vi "delta 0.1+7001.vi"() -> ()   [LabVIEW 2019]
uses:
  lib/Keithley 622x/Configure/Format/Typedefs/KE622x -- Results Format.ctl
  lib/Keithley 622x/Configure/Format/Typedefs/KE622x -- Optional Meas Elements.ctl
  lib/Keithley 622x/Configure/Delta PDelta DCon Modes/Typedefs/KE622x -- Delta Mode Params.ctl
  lib/Keithley 622x/Configure/Delta PDelta DCon Modes/Low Level/Typedefs/KE622x -- Delta PDelta Mode High Level.ctl
  lib/Keithley 622x/Configure/Delta PDelta DCon Modes/Low Level/Typedefs/KE622x -- Delta PDelta Mode Low Level.ctl
  lib/Keithley 622x/Configure/Delta PDelta DCon Modes/Low Level/Typedefs/KE622x -- Delta DCon Mode Delay.ctl
  lib/Keithley 622x/Configure/Delta PDelta DCon Modes/Low Level/Typedefs/KE622x -- Delta PDelta Mode Num Cycles Mode.ctl
  lib/Keithley 622x/Configure/Delta PDelta DCon Modes/Low Level/Typedefs/KE622x -- Delta PDelta Mode Num Cycles.ctl
  lib/Keithley 622x/Configure/2182 -A/Low Level/Typedefs/KE2182 -- Voltage Ranges.ctl
  lib/Keithley 622x/Configure/2182 -A/Low Level/Typedefs/KE2182 -- Filter Type.ctl
  lib/Keithley 622x/Configure/2182 -A/Low Level/Typedefs/KE2182 -- Filter Count.ctl
  lib/Keithley 622x/Configure/2182 -A/Low Level/Typedefs/KE2182 -- Filter Window.ctl
  lib/Keithley 622x/Configure/2182 -A/Low Level/Typedefs/KE2182 -- NPLCs.ctl
  lib/Keithley 622x/Configure/Units/Typedefs/KE622x -- Voltage Meas Units.ctl
  KE7001.LLB/Keith 7001 Open/Close Chan.vi
  <vilib>/Utility/file.llb/Write Delimited Spreadsheet (DBL).vi
  lib/Keithley 622x/Keithley 622x.lvlib
panel:
  in  "Meas Units":T1=enum."Ohms"
  out "XY图":cluster{dbl[], dbl[]}(graph)
  in  "file path (dialog if empty)":path caption="文件路径 （空时为对话框）"
  in  "622x Resource":refnum<visa-resource-name>
  in  "Check For SCPI Errors? (T)":bool=TRUE
  in  "2182/2182A Delta Mode Meas Params":T7={"Auto Range?"=TRUE, "Man / Selected\nRange"=enum."10mV", "Enable Digital\nFilter?"=FALSE, "Filter Type"=enum."Moving", "Filter Count"=10, "Filter\nWindow (%)"=0.01, "Enable Analog\nFilter?"=FALSE, "NPLCs"=5} {"Filter\nWindow (%)" min=0.0 max=10.0 step=0.01 format="%.2f"; "Filter Count" min=1 max=100; "NPLCs" min=1 max=10}
  in  "622x Delta Meas Mode Params":T8={"High Level (A)"=0.001, "Low Level (A)"=-0.001, "Delay (s)"=0.002, "Num Cycles Mode"=enum."Finite Count", "Finite Count"=10, "Abort On\nCompliance?"=FALSE, "Cold Swithing\nMode Enabled?"=FALSE} {"Finite Count" min=2 max=65536; "Low Level (A)" min=-0.105 max=0.0 format="%.3p"; "High Level (A)" min=0.0 max=0.105 format="%.3p"; "Delay (s)" min=0.001 max=9999.999 format="%.3f"}
  in  "Meas Timeout\n(msecs)":u32=20000
  out "Execution Time\n(secs)":dbl
  out "Meas\nTimeout?":bool
  in  "Meas Elements To Return":T14={"Timstamp?"=TRUE, "Reading Num?"=TRUE, "Source Value?"=TRUE, "Compliance?"=TRUE, "Average Voltage?"=TRUE}
  in  "Results Format":T15={"Results Format"=enum."Single Prec Bin", "Bin Byte Order"=enum."Swapped"}
  in  "Instrument Type":i32(ring)=3 items=["PPMS", "VersaLab", "DynaCool", "SVSM"]
  # "*** NOTE:  \"Average Voltage\"\nis only available for Differential\nConductance measurements."
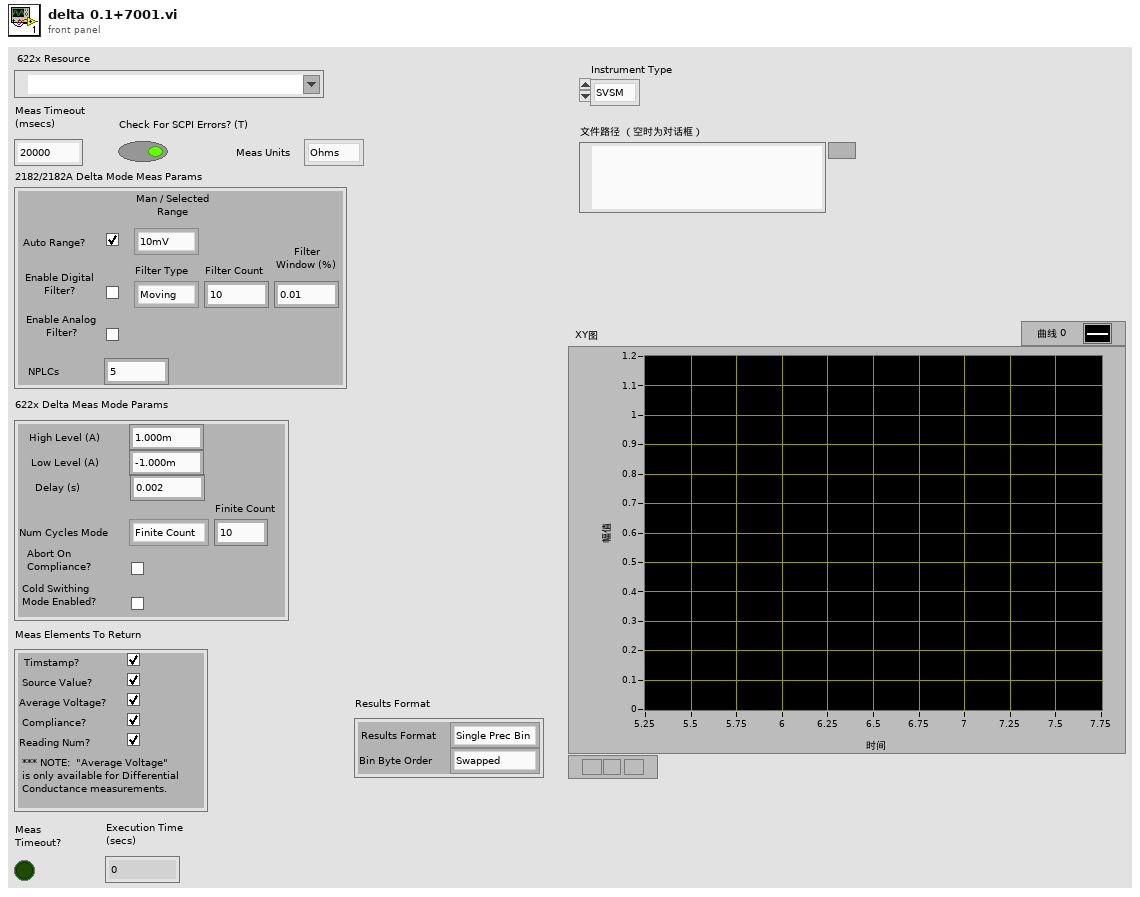
[diagram p1: front panel]
types:
  T1 = typedef "Keithley 622x.lvlib/KE622x -- Voltage Meas Units.ctl" = enum16{"Volts", "Ohms", "Watts", "Siemens"}
  T2 = typedef "Keithley 622x.lvlib/KE2182 -- Voltage Ranges.ctl" = enum16{"10mV", "100mV", "1V", "10V", "100V"}
  T3 = typedef "Keithley 622x.lvlib/KE2182 -- Filter Type.ctl" = enum16{"Moving", "Repeat"}
  T4 = typedef "Keithley 622x.lvlib/KE2182 -- Filter Count.ctl" = u32
  T5 = typedef "Keithley 622x.lvlib/KE2182 -- Filter Window.ctl" = dbl
  T6 = typedef "Keithley 622x.lvlib/KE2182 -- NPLCs.ctl" = u32
  T7 = cluster{"Auto Range?":bool, "Man / Selected\nRange":T2, "Enable Digital\nFilter?":bool, "Filter Type":T3, "Filter Count":T4, "Filter\nWindow (%)":T5, "Enable Analog\nFilter?":bool, "NPLCs":T6}
  T8 = typedef "Keithley 622x.lvlib/KE622x -- Delta Mode Params.ctl" = cluster{"High Level (A)":T9, "Low Level (A)":T10, "Delay (s)":T11, "Num Cycles Mode":T12, "Finite Count":T13, "Abort On\nCompliance?":bool, "Cold Swithing\nMode Enabled?":bool}
  T9 = typedef "Keithley 622x.lvlib/KE622x -- Delta PDelta Mode High Level.ctl" = dbl
  T10 = typedef "Keithley 622x.lvlib/KE622x -- Delta PDelta Mode Low Level.ctl" = dbl
  T11 = typedef "Keithley 622x.lvlib/KE622x -- Delta DCon Mode Delay.ctl" = dbl
  T12 = typedef "Keithley 622x.lvlib/KE622x -- Delta PDelta Mode Num Cycles Mode.ctl" = enum16{"Finite Count", "Infinite"}
  T13 = typedef "Keithley 622x.lvlib/KE622x -- Delta PDelta Mode Num Cycles.ctl" = u32
  T14 = typedef "Keithley 622x.lvlib/KE622x -- Optional Meas Elements.ctl" = cluster{"Timstamp?":bool, "Reading Num?":bool, "Source Value?":bool, "Compliance?":bool, "Average Voltage?":bool}
  T15 = typedef "Keithley 622x.lvlib/KE622x -- Results Format.ctl" = cluster{"Results Format":enum16{"ASCII", "Single Prec Bin", "Double Prec Bin"}, "Bin Byte Order":enum16{"Normal", "Swapped"}}
  T16 = enum16{"open", "replace", "create", "open or create", "replace or create", "replace or create with confirmation"}
  T17 = cluster{"slot/memory":i16, "channel/row":i16, "column":i16, bool, bool}[]
  T18 = cluster{"error":bool, "code":i32, "source":string}
  T19 = typedef "Keithley 622x.lvlib/KE622x -- Trace Buf.ctl" = cluster{"Additional Valid Arrays":T14, "Reading Num":u32[], "Timestamp (secs)":sgl[], "Source Val (A)":sgl[], "Reading":sgl[], "Average Voltage (V)":sgl[], "Compliance?":bool[]}
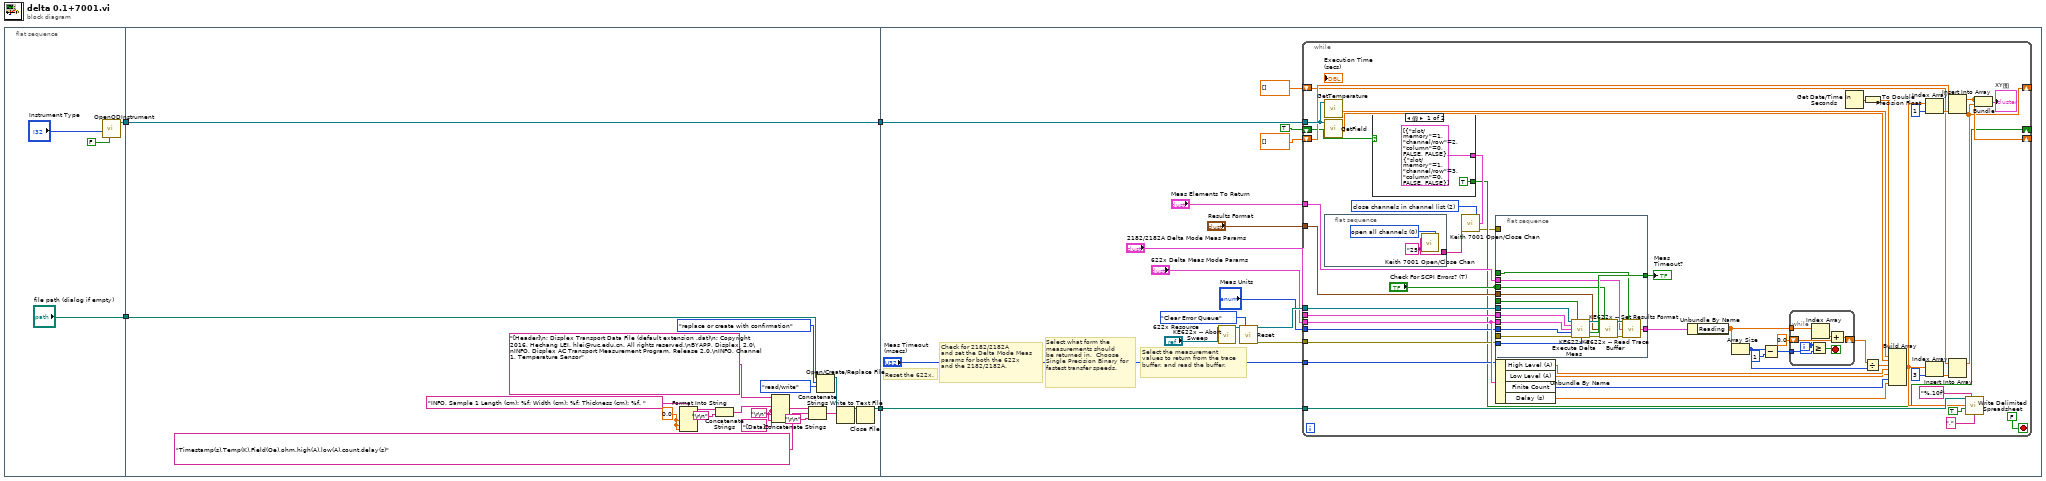
[diagram p0: block diagram]
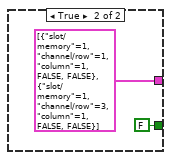
[diagram p2: hidden frame]
diagram:
  n1 = flat-sequence {
    tunnel: [w6] -> w4
    tunnel: ["file path (dialog if empty)"] -> w2
    tunnel: w4 -> [w27]
    tunnel: [w27] -> w3
    tunnel: w2 -> [w15]
    tunnel: [w10] -> w1
    tunnel: w3 -> [w43]
    tunnel: w1 -> [w34]
    frame #0 {
      n2 = call "OpenQDInstrument.vi"("Remote"=FALSE, "Instrument Type"="Instrument Type") -> ("Instrument Ref"=w6:refnum<k24>)  [unwired: 6 in, 1 out]
    }
    frame #1 {
      w22 = 0.0 ("输入 1")
      w19 = "\r\n"
      n3 = Format Into String(format string="INFO, Sample 1 Length (cm): %f; Width (cm): %f; Thickness (cm): %f. " ("string"), w22, w22, w22) -> (resulting string=w24:string)  [unwired: 2 in, 1 out]
      n4 = Concatenate Strings(w24, "\r\n") -> (w26:string)
      n5 = Concatenate Strings("[Header]\n; Displex Transport Data File (default extension .dat)\n; Copyright 2016, Hechang LEI, hlei@ruc.edu.cn. All rights reserved.\nBYAPP, Displex, 2.0\nINFO, Displex AC Transport Measurement Program, Release 2.0.\nINFO, Channel 1, Temperature Sensor" ("string"), w19, w26, w19, "[Data]" ("string"), w19) -> (w25:string)
      n6 = Concatenate Strings(w25, "Timestamp(s),Temp(K),Field(Oe),ohm,high(A),low(A),count,delay(s)" ("字符串"), "\r\n") -> (w16:string)
      n7 = Open/Create/Replace File(file path (use dialog)=w15, operation (0:open)=T16."replace or create with confirmation" ("操作(0:open)"), access (0:read/write)=enum16{"read/write", "read-only", "write-only"}."read/write" ("权限(0:read/write)")) -> (refnum out=w14:refnum<file>)  [unwired: 3 in, 2 out]
      n8 = Write to Text File(file (use dialog)=w14, text=w16) -> (refnum out=w11:refnum<file>)  [unwired: 2 in, 2 out]
      n9 = Close File(refnum=w11) -> (path=w10:path)  [unwired: 1 in, 1 out]
    }
    frame #2 {
      # "Select what form the\nmeasurements should\nbe returned in.  Choose\nSingle Precision Binary for\nfastest transfer speeds."
      # "Select the measurement\nvalues to return from the trace\nbuffer, and read the buffer."
      # "Check for 2182/2182A\nand set the Delta Mode Meas\nparams for both the 622x\nand the 2182/2182A."
      # "Reset the 622x."
      n10 = call "KE622x -- Abort Sweep.vi"("Resource In"="622x Resource") -> ("Resource Out (dupl)"=w30:refnum<visa-resource-name>)  [unwired: 13 in, 1 out]
      n11 = call "Reset.vi"("VISA resource name"=w30, "Error Queue Option"=enum16{"Clear Error Queue", "Error Query"}."Clear Error Queue") -> ("VISA resource name out"=w41:refnum<visa-resource-name>, "error out"=w38:errorcluster)  [unwired: 12 in]
      n12 = while {
        tunnel: w43 -> [w90]
        tunnel: w41 -> [w56]
        tunnel: "2182/2182A Delta Mode Meas Params" -> [w55]
        tunnel: "622x Delta Meas Mode Params" -> [w54]
        tunnel: "Meas Units" -> [w53]
        tunnel: w38 -> [w52]
        tunnel: "Meas Timeout\n(msecs)" -> [w51]
        tunnel: "Meas Elements To Return" -> [w47]
        tunnel: "Results Format" -> [w49]
        tunnel: w34 -> [w79]
        shift-right: [w64] -> _
        shift-left: T11[] [] -> [w67]
        shift-right: [w65] -> _
        shift-left: T11[] [] -> [w69]
        shift-right: [w45] -> _
        shift-left: TRUE -> [w57]
        stop <- FALSE stop-if-true
        w60 = u16 2 items=["open all channels", "open channels in channel list", "close channels in channel list"] ("open/close (open all:0)")
        n13 = call "GetTemperature.vi"("Instrument Ref In"=w90) -> ("Temperature"=w89:dbl)  [unwired: 4 in, 4 out]
        n14 = call "GetField.vi"("Instrument Ref In"=w90) -> ("Field"=w88:dbl)  [unwired: 4 in, 4 out]
        n15 = flat-sequence {
          tunnel: [w113] -> w59
          frame #0 {
            w114 = u16 0 items=["open all channels", "open channels in channel list", "close channels in channel list"] ("open/close (open all:0)")
            w113 = "25" ("GPIB address")
            n16 = call "Keith 7001 Open/Close Chan.vi"("GPIB address"=w113, "open/close (open all:0)"=w114) -> ()  [unwired: 2 in, 1 out]
          }
        }
        n17 = case shown="假" w57 {
          tunnel: [T17 [{"slot/memory"=1, "channel/row"=2, "column"=0, FALSE, FALSE}, {"slot/memory"=1, "channel/row"=3, "column"=0, FALSE, FALSE}] ("channel list") T17 [{"slot/memory"=1, "channel/row"=1, "column"=1, FALSE, FALSE}, {"slot/memory"=1, "channel/row"=3, "column"=1, FALSE, FALSE}] ("channel list")] -> w58
          tunnel: [TRUE FALSE] -> w45
          frame False {
          }
          frame True {
          }
        }
        n18 = call "Keith 7001 Open/Close Chan.vi"("GPIB address"=w59, "open/close (open all:0)"=w60, "channel list"=w58) -> ("error out"=w44:T18)  [unwired: 1 in]
        n19 = flat-sequence {
          tunnel: w56 -> [w108]
          tunnel: "Check For SCPI Errors? (T)" -> [w107]
          tunnel: w55 -> [w106]
          tunnel: w54 -> [w105]
          tunnel: w53 -> [w104]
          tunnel: w52 -> [w103]
          tunnel: w51 -> [w102]
          tunnel: [w101] -> w50
          tunnel: "Check For SCPI Errors? (T)" -> [w99]
          tunnel: w49 -> [w98]
          tunnel: "Check For SCPI Errors? (T)" -> [w95]
          tunnel: w47 -> [w94]
          tunnel: [w92] -> w46
          tunnel: w44 -> [_]
          frame #0 {
            n20 = call "KE622x -- Execute Delta Meas.vi"("Resource In"=w108, "Check For SCPI Errors? (T)"=w107, "2812 -A Params In"=w106, "Delta Mode Params In"=w105, "Meas Units"=w104, "error in (no error)"=w103, "Timeout (20000 ms)"=w102) -> ("Resource Out (dupl)"=w100:refnum<visa-resource-name>, "Timeout?"=w101:bool, "error out"=w97:errorcluster)  [unwired: 3 in, 3 out]
            n21 = call "KE622x -- Set Results Format.vi"("Resource In"=w100, "Check For SCPI Errors? (T)"=w99, "Results Format"=w98, "error in (no error)"=w97) -> ("Resource Out (dupl)"=w96:refnum<visa-resource-name>, "error out"=w93:errorcluster)  [unwired: 10 in]
            n22 = call "KE622x -- Read Trace Buffer.vi"("Resource In"=w96, "Check For SCPI Errors? (T)"=w95, "Meas Elements To Return"=w94, "error in (no error)"=w93) -> ("Trace Buf"=w92:T19)  [unwired: 9 in, 2 out]
          }
        }
        n23 = Unbundle By Name(w54) -> ("High Level (A)"=w76:T9, "Low Level (A)"=w75:T10, "Finite Count"=w74:T13, "Delay (s)"=w73:T11)
        n24 = Unbundle By Name(w46) -> ("Reading"=w84:sgl[])
        n25 = Array Size(array=w84) -> (size(s)=w61:i32)
        n26 = Subtract(x=w61, y=1) -> (x-y=w82:i32)
        n27 = while {
          tunnel: w84 -> [w121]
          shift-right: [w118] -> w86
          shift-left: sgl 0.0 ("Numeric") -> [w119]
          tunnel: w82 -> [w117]
          i -> [w116]
          stop <- w115 stop-if-true
          n28 = Greater Or Equal?(x=w116, y=w117) -> (x >= y?=w115:bool)
          n29 = Index Array(array=w121, index=w116) -> (element=w120:sgl)
          n30 = Add(x=w120, y=w119) -> (x+y=w118:sgl)
        }
        n31 = Get Date/Time In Seconds() -> (seconds since 1Jan1904=w78:timestamp)
        n32 = Divide(x=w86, y=w61) -> (x/y=w85:sgl)
        n33 = To Double Precision Float(number=w78) -> (double precision float=w77:dbl)
        n34 = Build Array(w77, w89, w88, w85, w76, w75, w74, w73) -> (w70:T11[])
        n35 = Index Array(array=w70, index=1 ("索引")) -> (element=w68:T11)
        n36 = Index Array(array=w70, index=3 ("索引")) -> (element=w66:T11)
        n37 = Insert Into Array(array=w69, new element=w68) -> (w65:T11[])  [unwired: 1 in]
        n38 = Insert Into Array(array=w67, new element=w66) -> (w64:T11[])  [unwired: 1 in]
        n39 = call-poly <vilib>:"Write Delimited Spreadsheet.vi"("file path (dialog if empty)"=w79, "format (%.3f)"="%.10f", "1D data"=w70, "append to file? (new file:F)"=TRUE, "delimiter (\\t)"="," ("delimiter (\\t)")) -> ()  [unwired: 9 in, 2 out]
        n40 = Bundle(w65, w64) -> (→"XY图":cluster{T11[], T11[]})  [unwired: 1 in]
        "Meas\nTimeout?" <- w50
      }
    }
  }
